vi "Cargo Arm Height.vi"(1 "Wanted Distance":dbl) -> (0 "Arm Final Speed":dbl)   [LabVIEW 2018]
uses:
  <vilib>/Rock Robotics/WPI/Utilities/WPI_GetSetVariantRefNum.vi
  Robot Global Data.vi
  <vilib>/addons/control/pid/pid.llb/PID (DBL).vi
  <vilib>/addons/control/pid/NI_PID_pid.lvlib
panel:
  in  "Range":cluster{"MAX":dbl, "MIN":dbl}={"MAX"=0.75, "MIN"=-0.75}
  in  "PID Gains":cluster{"P":dbl, "I":dbl, "D":dbl}
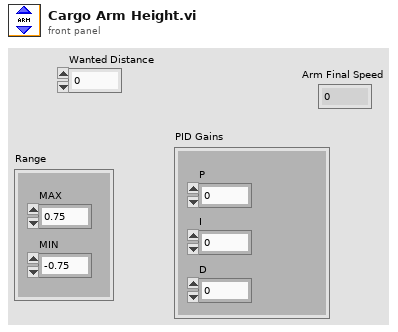
[diagram p1: front panel]
types:
  T1 = typedef "WPI_JoystickDevRef.ctl" = cluster{"Device":T2}
  T2 = typedef "WPI_JoystickDeviceEnum.ctl" = enum16{"USB 0", "USB 1", "USB 2", "USB 3", "USB 4", "USB 5"}
  T3 = typedef "WPI_EncoderDevRef.ctl" = cluster{"DevStatus":errorcluster, "EncoderIndex":T4, "CounterIndex":T5, "DistancePerCount":dbl, "Decoding Type":T6}
  T4 = typedef "FPGA_EncoderIdx.ctl" = enum8{"Enc 0", "Enc 1", "Enc 2", "Enc 3", "Enc 4", "Enc 5", "Enc 6", "Enc 7", "Invalid"}
  T5 = typedef "FPGA_CounterCtrSystemIndex.ctl" = enum8{"Ctr 0", "Ctr 1", "Ctr 2", "Ctr 3", "Ctr 4", "Ctr 5", "Ctr 6", "Ctr 7", "Invalid"}
  T6 = typedef "WPI_EncoderType.ctl" = enum16{"1x", "2x", "4x"}
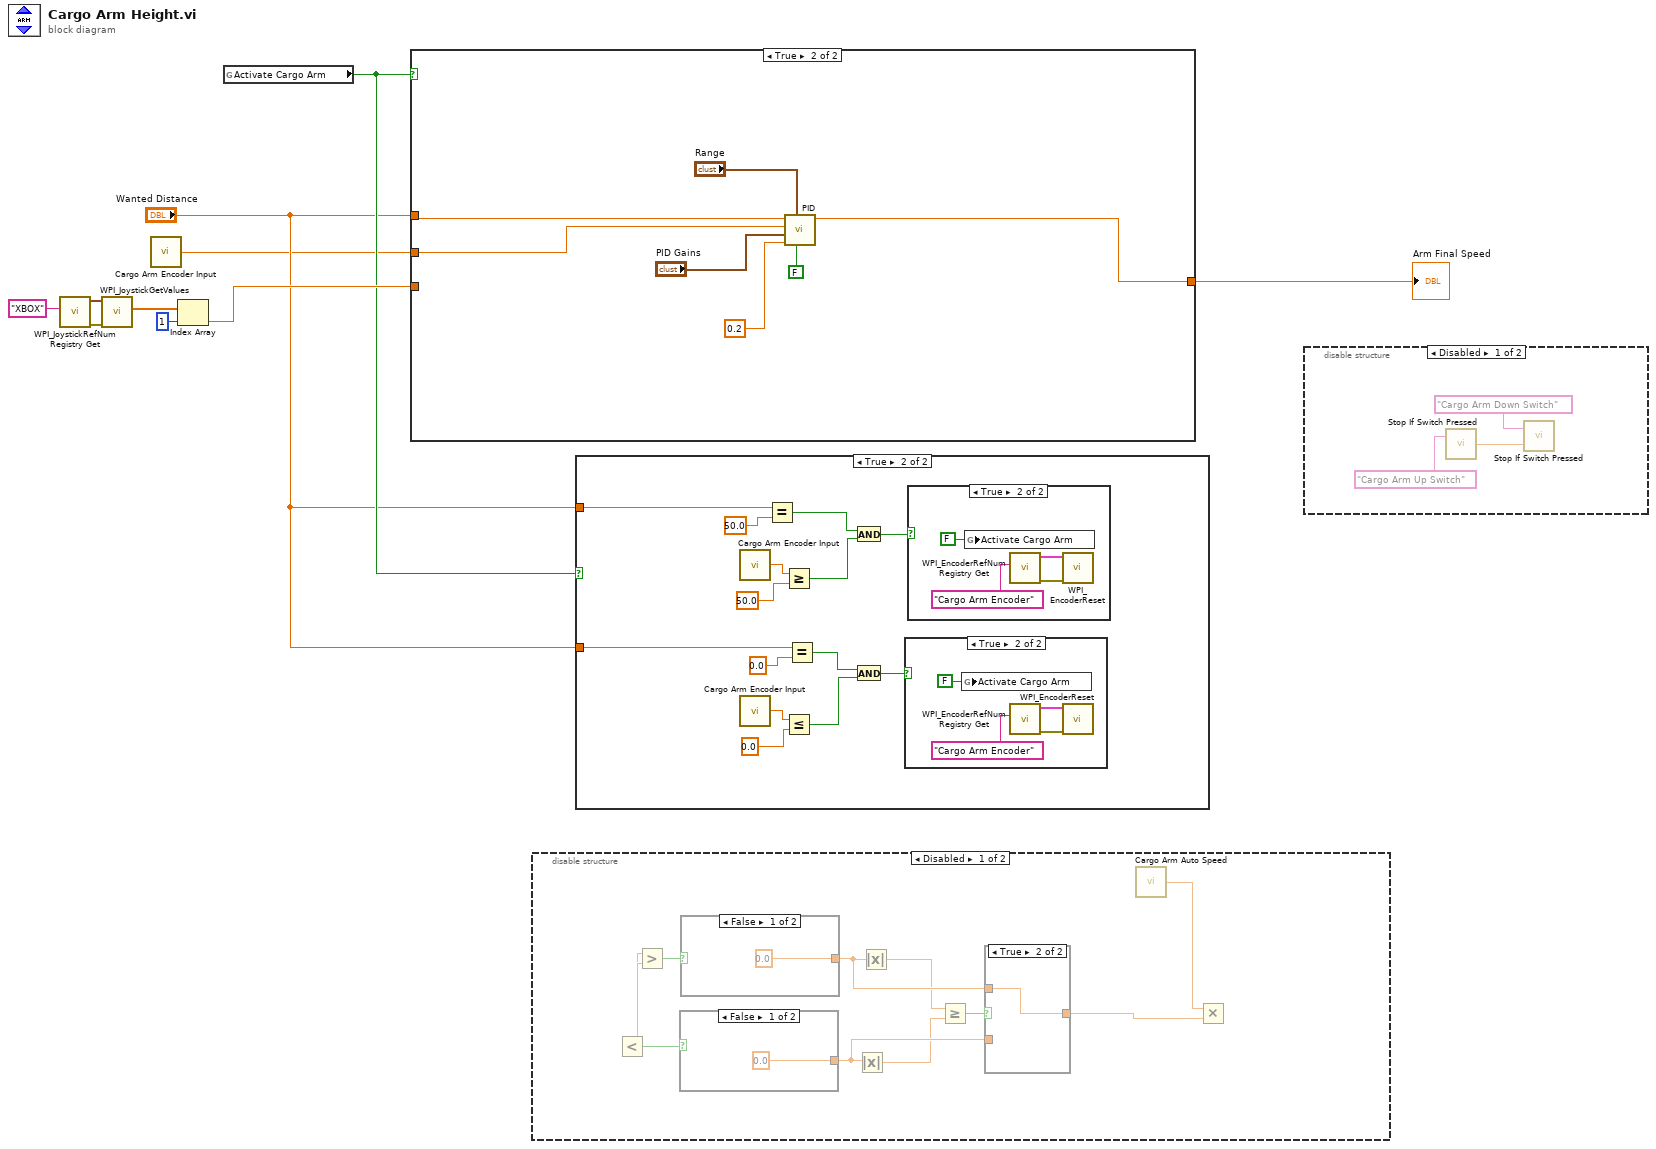
[diagram p0: block diagram]
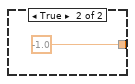
[diagram p3: hidden frame]
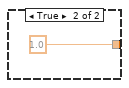
[diagram p4: hidden frame]
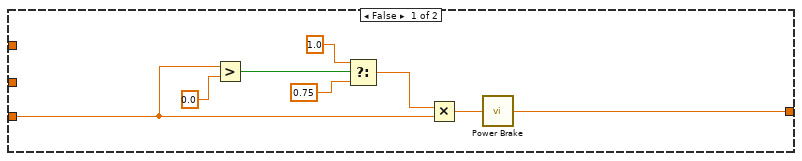
[diagram p10: hidden frame]
diagram:
  n1 = call <vilib>:"WPI_JoystickRefNum Registry Get.vi"("refnum name"="XBOX") -> ("error out"=w10:errorcluster, "JoystickDevRef"=w9:T1)  [unwired: 9 in]
  n2 = call <vilib>:"WPI_JoystickGetValues.vi"("error in (no error)"=w10, "JoystickDevRef"=w9) -> ("Axes"=w7:dbl[])  [unwired: 5 in, 4 out]
  n3 = call "Cargo Arm Encoder Input.vi"() -> ("Cargo Arm Distance (cm)"=w2:dbl)  [unwired: 1 in]
  n4 = Index Array(array=w7, index=1) -> (element=w5:dbl)
  n5 = global read "Robot Global Data.vi" "Activate Cargo Arm"() -> (w4:bool)
  n6 = case shown="True" w4 {
    tunnel: "Wanted Distance" -> [_ w25]
    tunnel: w2 -> [_ w19]
    tunnel: [w11 w24] -> w1
    tunnel: w5 -> [w16 _]
    frame False {
      n7 = Greater?(x=w16, y=0.0) -> (0:w13:bool)
      n8 = Select(t=1.0, s=w13, f=0.75) -> (s? t:f=w14:dbl)
      n9 = Multiply(x=w14, y=w16) -> (x*y=w12:dbl)
      n10 = call "Power Brake.vi"("Arm Speed"=w12) -> ("Final Speed Value"=w11:dbl)
    }
    frame True {
      n11 = call-poly <vilib>:"PID.vi"("reinitialize? (F)"=FALSE, "output range"="Range", "dt (s)"=0.2, "PID gains"="PID Gains", "process variable"=w19, "setpoint"=w25) -> ("output"=w24:dbl)  [unwired: 4 in, 1 out]
    }
  }
  "Arm Final Speed" <- w1
  n12 = disable-structure shown="Disabled" {
    frame Disabled {
      n13 = call "Cargo Arm Auto Speed.vi"() -> ("Final Speed"=w29:dbl, "Current Distance (x)"=w27:dbl)
      n14 = Less?(y=w33) -> (x=w32:dbl, x < y?=w30:bool)
      n15 = Greater?(x=w32) -> (y=w33:dbl, 0:w31:bool)
      n16 = case shown="False" w30 {
        tunnel: [0.0 -1.0] -> w37
        frame False {
        }
        frame True {
        }
      }
      n17 = case shown="False" w31 {
        tunnel: [0.0 1.0] -> w35
        frame False {
        }
        frame True {
        }
      }
      n18 = Absolute Value(x=w37) -> (abs(x)=w36:dbl)
      n19 = Absolute Value(x=w35) -> (abs(x)=w34:dbl)
      n20 = Greater Or Equal?(x=w34, y=w36) -> (x >= y?=w38:bool)
      n21 = case shown="True" w38 {
        tunnel: [w39 w40] -> w26
        tunnel: w35 -> [_ w40]
        tunnel: w37 -> [w39 _]
        frame False {
        }
        frame True {
        }
      }
      n22 = Multiply(x=w29, y=w26) -> (x*y=w28:dbl)
    }
    frame Enabled {
    }
  }
  n23 = case shown="True" w4 {
    tunnel: "Wanted Distance" -> [_ w53]
    tunnel: "Wanted Distance" -> [_ w45]
    frame False {
    }
    frame True {
      n24 = call "Cargo Arm Encoder Input.vi"() -> ("Cargo Arm Distance (cm)"=w58:dbl)  [unwired: 1 in]
      n25 = call "Cargo Arm Encoder Input.vi"() -> ("Cargo Arm Distance (cm)"=w56:dbl)  [unwired: 1 in]
      n26 = Equal?(x=w53, y=50.0) -> (x = y?=w51:bool)
      n27 = Greater Or Equal?(x=w58, y=50.0) -> (x >= y?=w52:bool)
      n28 = Less Or Equal?(x=w56, y=0.0) -> (x <= y?=w49:bool)
      n29 = Equal?(x=w45, y=0.0) -> (x = y?=w46:bool)
      n30 = And(x=w51, y=w52) -> (x .and. y?=w50:bool)
      n31 = And(x=w46, y=w49) -> (x .and. y?=w48:bool)
      n32 = case shown="True" w48 {
        frame False {
        }
        frame True {
          n33 = global write "Robot Global Data.vi" "Activate Cargo Arm"(FALSE ("Activate Cargo Arm")) -> ()
          n34 = call <vilib>:"WPI_EncoderRefNum Registry Get.vi"("refnum name"="Cargo Arm Encoder") -> ("error out"=w61:errorcluster, "EncoderDevRef"=w60:T3)  [unwired: 9 in]
          n35 = call <vilib>:"WPI_EncoderReset.vi"("error in (no error)"=w61, "EncoderDevRef"=w60) -> ()  [unwired: 8 in, 2 out]
        }
      }
      n36 = case shown="True" w50 {
        frame False {
        }
        frame True {
          n37 = global write "Robot Global Data.vi" "Activate Cargo Arm"(FALSE ("Activate Cargo Arm")) -> ()
          n38 = call <vilib>:"WPI_EncoderRefNum Registry Get.vi"("refnum name"="Cargo Arm Encoder") -> ("error out"=w65:errorcluster, "EncoderDevRef"=w64:T3)  [unwired: 9 in]
          n39 = call <vilib>:"WPI_EncoderReset.vi"("error in (no error)"=w65, "EncoderDevRef"=w64) -> ()  [unwired: 8 in, 2 out]
        }
      }
    }
  }
  n40 = disable-structure shown="Disabled" {
    frame Disabled {
      n41 = call "Stop If Switch Pressed.vi"("Switch Name"="Cargo Arm Up Switch") -> ("Motor Value"=w67:dbl)  [unwired: 1 in]
      n42 = call "Stop If Switch Pressed.vi"("Motor Original Value"=w67, "Switch Name"="Cargo Arm Down Switch") -> ()  [unwired: 1 out]
    }
    frame Enabled {
    }
  }
